vi "Open.vi"(8 "error in (no error)":errorcluster, 10 "Update Rate (4Hz-100Hz)":u8=100, 11 "navX - SERIAL in":refnum<class "navX - SERIAL.lvclass">) -> (0 "error out":errorcluster, 3 "navX - SERIAL out":refnum<class "navX - SERIAL.lvclass">)   [LabVIEW 2015, in "navX Library v3.lvlib" / "navX - SERIAL.lvclass"]
uses:
  navX - SERIAL.lvclass
  _NI WPI Serial USB/WPI_SerialPort_USB.ctl
  navX - SERIAL.lvclass/navX - SERIAL.ctl
  navX - Interface/navX - Interface.lvclass
  _NI WPI Serial USB/_NI WPI Serial USB.lvlib
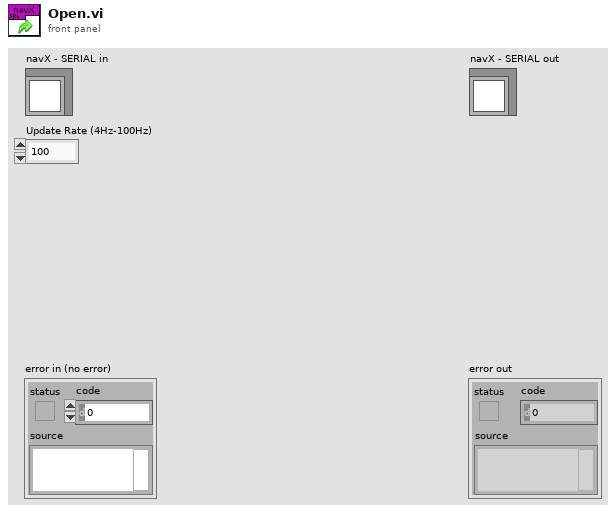
[diagram p1: front panel]
types:
  T1 = typedef "_NI WPI Serial USB.lvlib/WPI_SerialPort_USB.ctl" = enum16{"Onboard RS-232", "MXP TTL", "USB"}
  T2 = typedef "WPI_SerialPortRef.ctl" = cluster{"DevStatus":errorcluster, "Serial Port Name":refnum<visa-resource-name>}
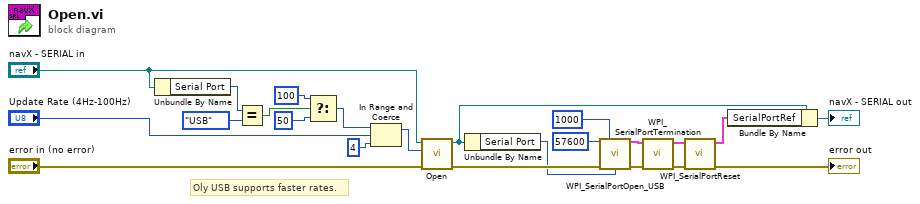
[diagram p0: block diagram]
diagram:
  # "Oly USB supports faster rates."
  n1 = Unbundle By Name("navX - SERIAL in") -> ("Serial Port"=w10:T1)
  n2 = Equal?(x=w10, y=WPI_SerialPort_USB."USB") -> (x = y?=w8:bool)
  n3 = Select(t=u8 100, s=w8, f=u8 50) -> (s? t:f=w3:u8)
  n4 = In Range and Coerce(upper limit=w3, x="Update Rate (4Hz-100Hz)", lower limit=u8 4) -> (coerced(x)=w1:u8)  [unwired: 1 out]
  n5 = call-parent "Open.vi"("error in (no error)"="error in (no error)", "Update Rate (4Hz-100Hz)"=w1, "navX - Interface in"="navX - SERIAL in") -> ("error out"=w16:errorcluster, "navX - Interface out"=w14:refnum<class "navX - SERIAL.lvclass">)  [unwired: 7 in]
  n6 = Unbundle By Name(w14) -> ("Serial Port"=w15:T1)
  n7 = call "WPI_SerialPortOpen_USB.vi"("Baud Rate"=u32 57600, "Timeout Value (ms)"=u32 1000, "error in (no error)"=w16, "Serial Port"=w15) -> ("SerialPortRef"=w19:T2, "error out"=w20:errorcluster)  [unwired: 10 in]
  n8 = call <vilib>:"WPI_SerialPortTermination.vi"("error in (no error)"=w20, "SerialPortRef"=w19) -> ("error out"=w18:errorcluster, "SerialPortRef"=w17:T2)  [unwired: 8 in]
  n9 = call <vilib>:"WPI_SerialPortReset.vi"("error in (no error)"=w18, "SerialPortRef"=w17) -> ("error out"=→"error out":errorcluster, "SerialPortRef"=w12:T2)  [unwired: 8 in]
  n10 = Bundle By Name(cluster=w14, "SerialPortRef"=w12) -> (→"navX - SERIAL out":refnum<class "navX - SERIAL.lvclass">)
